vi "IPC.vi"   [LabVIEW 2014]
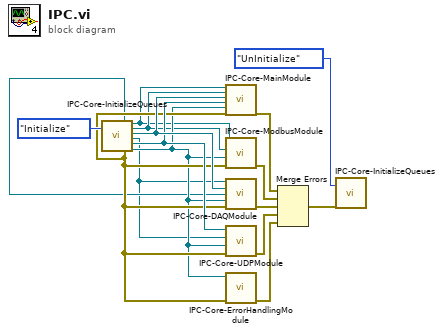
[diagram p0: block diagram]
diagram:
  n1 = call "IPC-Core-InitializeQueues.vi"("comand (Initialize)"=enum16{"UnInitialize", "Initialize"}."Initialize") -> ("6133QRef"=w2:refnum<queue>, "error out"=w11:errorcluster, "CmdQRef"=w3:refnum<queue>, "ModbusQRef"=w4:refnum<queue>, "DaqQRef"=w15:refnum<queue>, "DataQRef"=w1:refnum<queue>, "UdpQRef"=w12:refnum<queue>, "ErrorQRef"=w5:refnum<queue>)  [unwired: 11 in]
  n2 = call "IPC-Core-MainModule.vi"("CmdQRef"=w3, "ModbusQRef"=w4, "DaqQRef"=w15, "UdpQRef"=w12, "ErrorQRef"=w5, "error in"=w11) -> ("error out"=w6:errorcluster)  [unwired: 13 in]
  n3 = call "IPC-Core-ModbusModule.vi"("error in"=w11, "ErrorQRef"=w5, "ModbusQRef"=w4, "CmdQRef"=w3) -> ("error out"=w7:errorcluster)  [unwired: 7 in]
  n4 = call "IPC-Core-DAQModule.vi"("DataQRef"=w1, "DaqQRef"=w15, "6133QRef"=w2, "ErrorQRef"=w5, "error in"=w11) -> ("错误输出"=w8:errorcluster)  [unwired: 10 in]
  n5 = call "IPC-Core-UDPModule.vi"("error in"=w11, "ErrorQRef"=w5, "DataQRef"=w1, "UdpQRef"=w12) -> ("错误输出"=w14:errorcluster)  [unwired: 7 in]
  n6 = call "IPC-Core-ErrorHandlingModule.vi"("error in"=w11, "ErrorQRef"=w5) -> ("error out"=w13:errorcluster)  [unwired: 9 in]
  n7 = Merge Errors(w6, w7, w8, w14, w13) -> (w9:errorcluster)
  n8 = call "IPC-Core-InitializeQueues.vi"("comand (Initialize)"=enum16{"UnInitialize", "Initialize"}."UnInitialize", "error in (no error)"=w9) -> ()  [unwired: 10 in, 8 out]
